vi "FTW-JSON-KeyExists.vi"(0 "JSON Object":refnum<class "FTW-Container.lvclass">, 5 "Key":string, 11 "error in":errorcluster) -> (4 "JSON Object":refnum<class "FTW-Container.lvclass">, 6 "Found?":bool, 15 "error out":errorcluster)   [LabVIEW 2015]
uses:
  container/FTW-Container.lvclass
panel:
  # "Inputs"
  # "Outputs"
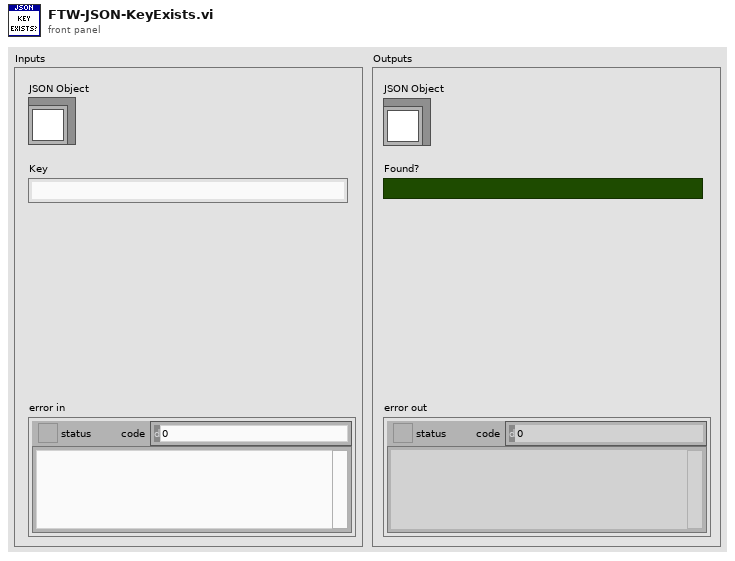
[diagram p1: front panel]
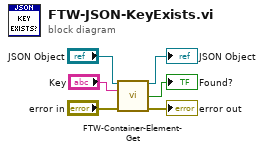
[diagram p0: block diagram]
diagram:
  n1 = call "FTW-Container-Element-Get.vi"("FTW-Container In"="JSON Object", "Element Name"="Key", "error in"="error in") -> ("FTW-Container Out"=→"JSON Object":refnum<class "FTW-Container.lvclass">, "Found"=→"Found?":bool, "error out"=→"error out":errorcluster)  [unwired: 9 in, 1 out]
